vi "Create Numeric Constant.vi"(5 "Sink":refnum<vi>, 6 "relative position/next to refnum":T1, 8 "error in (no error)":errorcluster, 10 "Value":variant, 11 "Diagram":refnum<vi>) -> (0 "error out":errorcluster, 2 "Output Terminal":refnum<vi>, 3 "Constant Ref":refnum<vi>)   [LabVIEW 2012, in "Scripting Tools.lvlib"]
uses:
  Scripting Tools.lvlib
  <vilib>/Utility/miscctls.llb/LVPointTypeDef.ctl
  <vilib>/Utility/VariantDataType/VariantType.lvlib
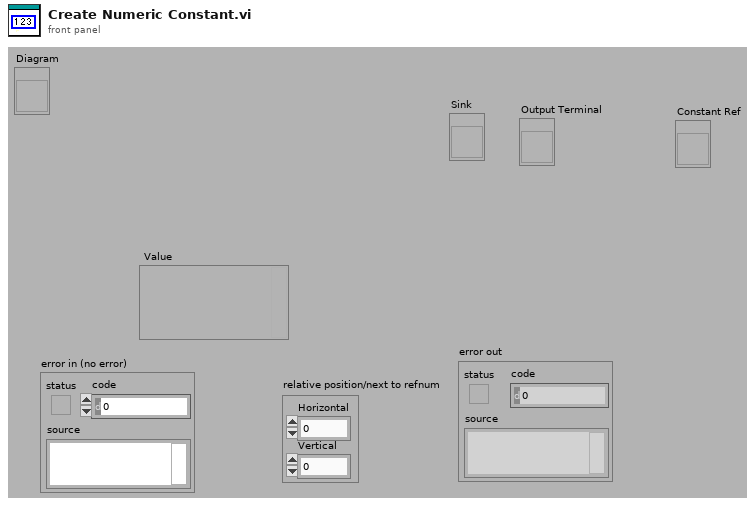
[diagram p1: front panel]
types:
  T1 = typedef "LVPointTypeDef.ctl" = cluster{"Horizontal":i16, "Vertical":i16}
  T2 = typedef "VariantType.lvlib/Type.ctl" = enum8{"Invalid Type", "Void", "I8", "I16", "I32", "I64", "U8", "U16", "U32", "U64", "Single Float", "Double Float", "Extended Float", "Single Complex", "Double Complex", "Extended Complex", "Enum U8", "Enum U16", "Enum U32", "Enum U64", "Single Float With Unit", "Double Float With Unit", "Extended Float With Unit", "Single Complex with Unit", "Double Complex with Unit", "Extended Complex with Unit", "Boolean", "String", "Path", "Picture", "Tag", "Array", "Cluster", "Variant", "LV Variant", "Waveform", "Timestamp", "Digital Waveform", "Digital Data", "ExpressData", "Refnum", "External Data", "VI", "Poly VI", "LabVIEW Class Instance", "Fixed Point"}
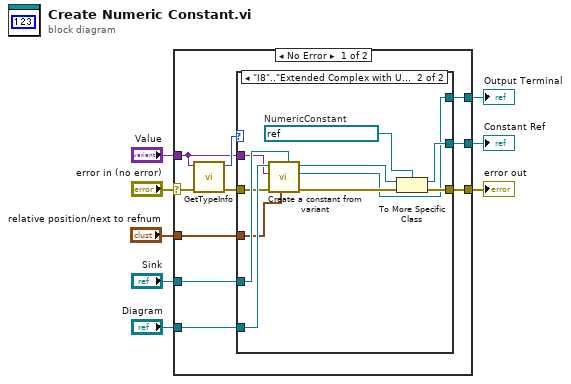
[diagram p0: block diagram]
diagram:
  n1 = case shown="No Error" "error in (no error)" {
    selector: "error in (no error)" -> [w18 w31]
    tunnel: "Diagram" -> [w16 _]
    tunnel: [w13 w31] -> w8
    tunnel: "Value" -> [w9 _]
    tunnel: "Sink" -> [w15 _]
    tunnel: [w12 _] -> w3
    tunnel: [w11 _] -> w2
    tunnel: "relative position/next to refnum" -> [w10 _]
    frame No Error {
      n2 = call <vilib>:"GetTypeInfo.vi"("error in (no error)"=w18, "Variant"=w9) -> ("error out"=w14:errorcluster, "Type Enum"=w17:T2)  [unwired: 8 out]
      n3 = case shown="\"I8\"..\"Extended Complex with Unit\"" w17 {
        tunnel: w16 -> [_ w30]
        tunnel: w15 -> [_ w29]
        tunnel: w10 -> [_ w28]
        tunnel: w14 -> [w19 w27]
        tunnel: [w19 w24] -> w13
        tunnel: [_ w23] -> w12
        tunnel: [_ w21] -> w11
        tunnel: w9 -> [_ w20]
        frame "Invalid Type", Default {
        }
        frame "I8".."Extended Complex with Unit" {
          w22 = refnum<vi> refnum  # NumericConstant
          n4 = call <userlib>:"Create a constant from variant.vi"("Terminal Sink"=w29, "relative position/next to refnum"=w28, "error in (no error)"=w27, "Constant Data"=w20, "Diagram"=w30) -> ("error out"=w25:errorcluster, "Terminal"=w21:refnum<vi>, "Const Refnum"=w26:refnum<vi>)  [unwired: 4 out]
          n5 = To More Specific Class(target class=w22, reference=w26, error in=w25) -> (specific class reference=w23:refnum<vi>, error out=w24:errorcluster)
        }
      }
    }
    frame Error {
    }
  }
  "Output Terminal" <- w2
  "error out" <- w8
  "Constant Ref" <- w3
